vi "Derivative x(t) PtByPt.vi"(2 "initialize":bool, 3 "dt":dbl=1.0 format="%0.2f", 4 "initial condition":dbl format="%0.2f", 5 "x":dbl format="%0.2f") -> (0 "error":i32, 1 "dx/dt":dbl format="%0.2f")   [LabVIEW 2020, in "NI_PtbyPt.lvlib"]
doc: "Performs a discrete differentiation on <B>x</B>."
uses:
  <vilib>/ptbypt/NI_PtbyPt.lvlib
  <vilib>/Analysis/NI_AALPro.lvlib
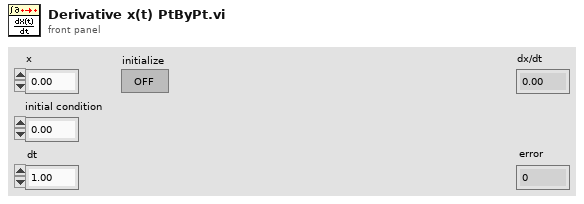
[diagram p1: front panel]
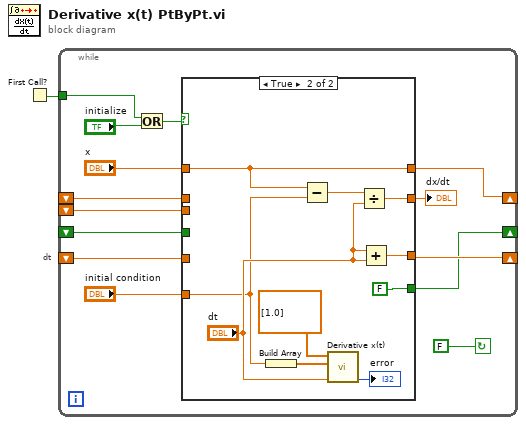
[diagram p0: block diagram]
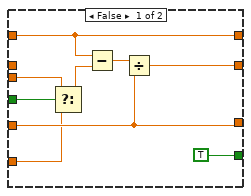
[diagram p2: hidden frame]
diagram:
  # "dt"
  n1 = First Call?() -> (First Call?: T/F=w1:bool)
  n2 = while {
    shift-left: _ -> [w4]
    shift-right: [w5] -> _
    shift-left: _ -> [w8]
    shift-right: [w11] -> _
    tunnel: w1 -> [w14]
    shift-left: _ -> [w7]
    shift-left: _ -> [w3]
    shift-right: [w6] -> _
    stop <- FALSE continue-if-true
    n3 = Or(x=w14, y="initialize") -> (x .or. y?=w12:bool)
    n4 = case shown="True" w12 {
      tunnel: [w22 w30] -> w11
      tunnel: "x" -> [w23 w32]
      tunnel: [w24 w33] -> w9
      tunnel: w8 -> [w22 _]
      tunnel: w7 -> [w18 _]
      tunnel: [w23 w32] -> w6
      tunnel: [TRUE FALSE] -> w5
      tunnel: w4 -> [w19 _]
      tunnel: w3 -> [_ _]
      tunnel: "initial condition" -> [w17 w26]
      frame False {
        n5 = Select(t=w18, s=w19, f=w17) -> (s? t:f=w16:dbl)
        n6 = Subtract(x=w23, y=w16) -> (x-y=w20:dbl)
        n7 = Divide(x=w20, y=w22) -> (x/y=w24:dbl)
      }
      frame True {
        n8 = Build Array(w26) -> (w25:dbl[])
        n9 = Subtract(x=w32, y=w26) -> (x-y=w34:dbl)
        n10 = call <vilib>:"Derivative x(t).vi"("dt"="dt", "Initial Condition"=w25, "X"=dbl[] [1.0]) -> ("error"=→"error":i32)  [unwired: 7 in, 1 out]
        n11 = Divide(x=w34, y="dt") -> (x/y=w33:dbl)
        n12 = Add(x="dt", y="dt") -> (x+y=w30:dbl)
      }
    }
    "dx/dt" <- w9
  }
